vi "Read_Camera.vi"(0 "error in":errorcluster, 2 "Camera":T2, 3 "node":string) -> (1 "error out":errorcluster, 4 "image out":T3 {"Dialogs" format="%.0b"})   [LabVIEW 2010]
doc: "Get an image from one of Baxter's hand cameras. \n\nIt is highly recommended that you are connected to baxter via ethernet rather than over wireless when doing this."
uses:
  <userlib>/ImageProcessing/QTLIB_2595_LV86/QT_Image.ctl
  <userlib>/ROSforLV_0.1/ROS/Code/SubVIs/BaxterCamera.ctl
panel:
  out "ROS Image":T1
  out "image":picture
  out "Reply":string
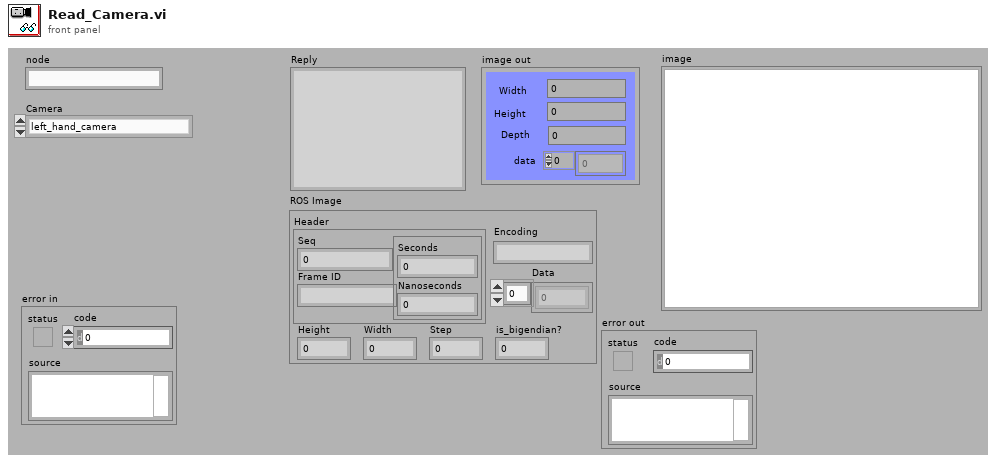
[diagram p1: front panel]
types:
  T1 = cluster{"Header":cluster{"Seq":u32, "Frame ID":string, cluster{"Seconds":i32, "Nanoseconds":i32}}, "Height":u32, "Width":u32, "is_bigendian?":u8, "Step":u32, "Data":u8[], "Encoding":string}
  T2 = typedef "BaxterCamera.ctl" = enum16{"left_hand_camera", "right_hand_camera", "head_camera"}
  T3 = typedef "QT_Image.ctl" = cluster{"Width":i32, "Height":i32, "Depth":i32, "data":u8[], "Compressed data":u8[], "Color table":u32[], "Duration":i32, "Options":i32, "Timestamp":i32, "ID":i32, "Reserved":i32, "Dialogs":u32}
  T4 = typedef "_ROSControl.ctl" = cluster{"topic port":u16, "Node":string, "topic":string, "type":string, "node port":u32, "error ":errorcluster, "Direction":T5, "APIs":string[]}
  T5 = typedef "_ROSDirection.ctl" = enum16{"Node", "Publisher", "Subscriber", "Service Client"}
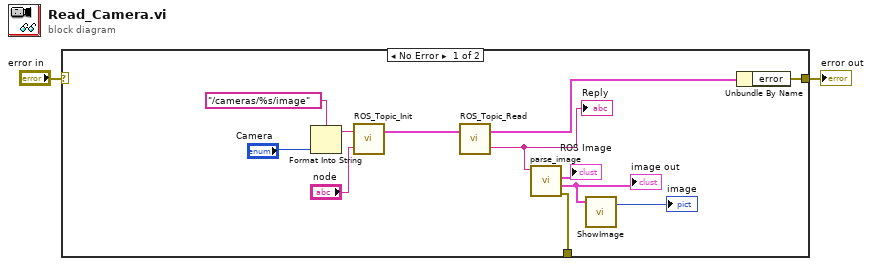
[diagram p0: block diagram]
diagram:
  n1 = case shown="No Error" "error in" {
    selector: "error in" -> [_ w15]
    tunnel: [w14 w15] -> w2
    tunnel: [w6 _] -> _
    frame No Error {
      n2 = Format Into String(format string="/cameras/%s/image" ("topic"), "Camera") -> (resulting string=w9:string)  [unwired: 2 in, 1 out]
      n3 = call <userlib>:"ROS_Topic_Init.vi"("node"="node", "topic"=w9) -> ("ROS out"=w12:T4)  [unwired: 1 in]
      n4 = call <userlib>:"ROS_Topic_Read.vi"("ROS in"=w12) -> ("Reply"=w8:string, "ROS out"=w11:T4)  [unwired: 1 in]
      "Reply" <- w8
      n5 = call <userlib>:"parse_image.vi"("msg in"=w8) -> ("error out"=w6:errorcluster, "Image Out"=w5:T3, "ROS Image"=→"ROS Image":T1)  [unwired: 3 in, 1 out]
      "image out" <- w5
      n6 = call <userlib>:"ShowImage.vi"("Image"=w5) -> ("image"=→"image":picture)  [unwired: 2 in, 1 out]
      n7 = Unbundle By Name(w11) -> ("error"=w14:errorcluster)
    }
    frame Error {
    }
  }
  "error out" <- w2
